vi "Start Experiment Set.vi"(8 "error in (no error)":errorcluster, 11 "ExperimentService in":refnum<class "ExperimentService.lvclass">) -> (0 "error out":errorcluster, 3 "ExperimentService out":refnum<class "ExperimentService.lvclass">)   [LabVIEW 2014, in "ExperimentService.lvclass"]
uses:
  ExperimentService.lvclass
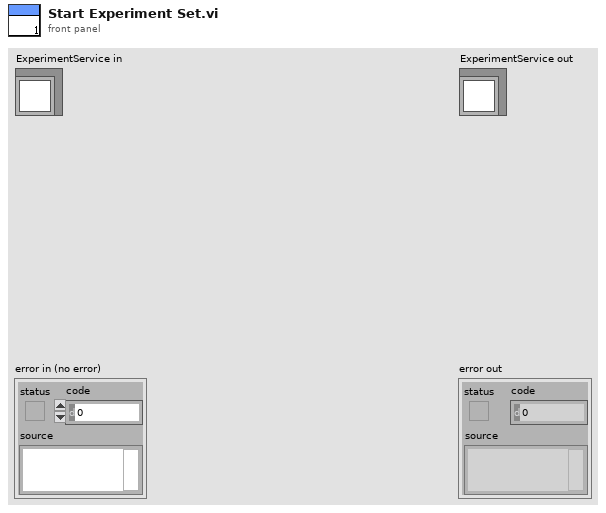
[diagram p1: front panel]
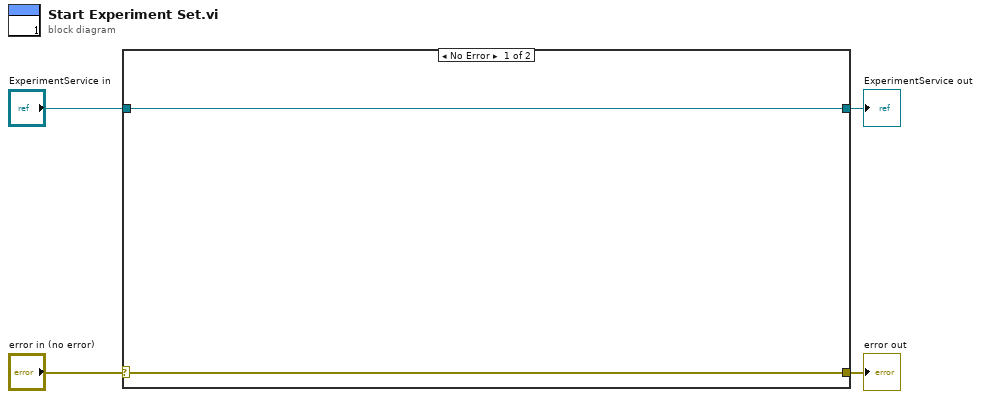
[diagram p0: block diagram]
diagram:
  n1 = case shown="No Error" "error in (no error)" {
    selector: "error in (no error)" -> [w6 w8]
    tunnel: [w6 w8] -> w3
    tunnel: [w5 w7] -> w1
    tunnel: "ExperimentService in" -> [w5 w7]
    frame No Error {
    }
    frame Error {
    }
  }
  "error out" <- w3
  "ExperimentService out" <- w1
